vi "Velmex cfg simulation.vi"(8 "error in (no error)":errorcluster {"code" format="%.0x"}, 10 "Channel parsed command info":T1, 11 "input cluster":refnum<class "VelmexStage.lvclass">) -> (0 "error out":errorcluster, 2 "new commands":string, 3 "output cluster":refnum<class "VelmexStage.lvclass">)   [LabVIEW 2013, in "VelmexStage.lvclass"]
uses:
  VelmexStage.lvclass
  channel parsed cmd cluster.ctl
  VelmexStage.lvclass/VelmexStage.ctl
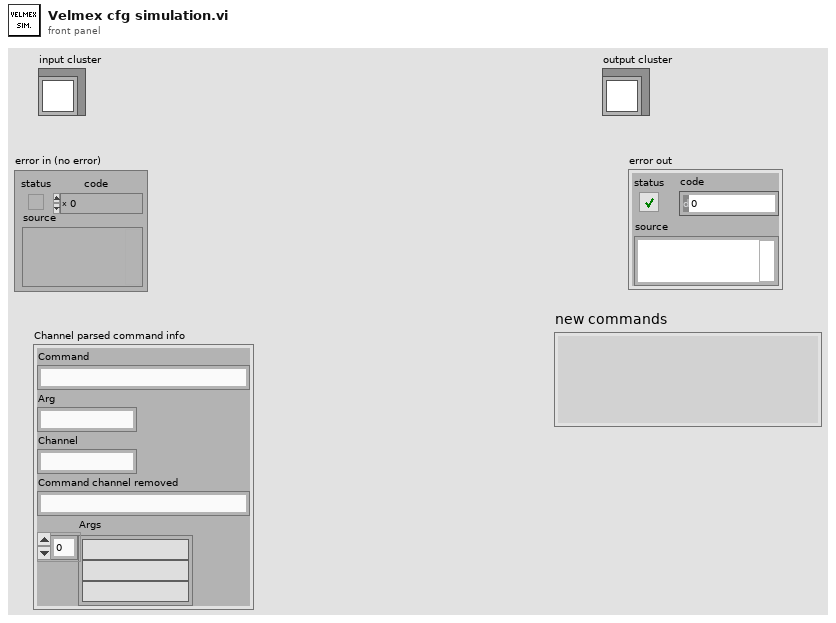
[diagram p1: front panel]
types:
  T1 = typedef "channel parsed cmd cluster.ctl" = cluster{"Command":string, "Arg":string, "Channel":string, "Command channel removed":string, "Args":string[]}
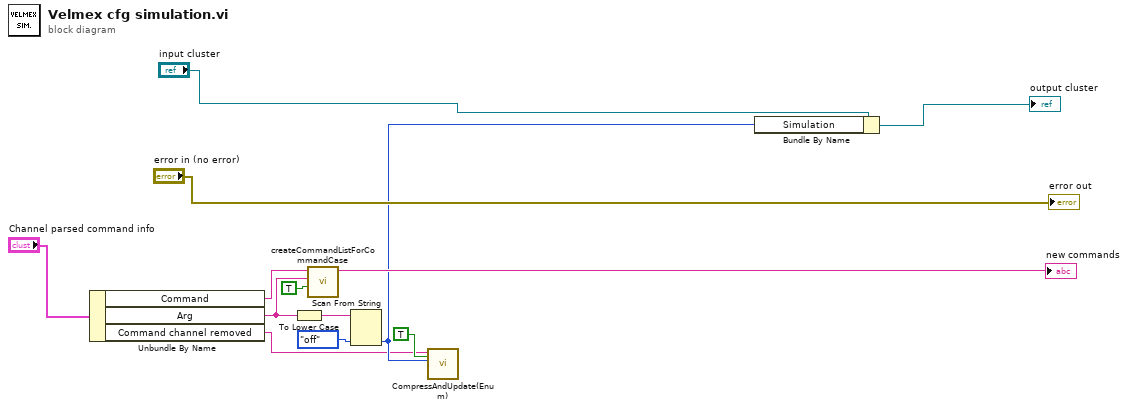
[diagram p0: block diagram]
diagram:
  n1 = Unbundle By Name("Channel parsed command info") -> ("Command"=w2:string, "Arg"=w5:string, "Command channel removed"=w1:string)
  n2 = To Lower Case(string=w5) -> (all lower case string=w7:string)
  n3 = call "createCommandListForCommandCase.vi"("immediate Check (only once)"=TRUE, "setvalue"=w5, "command"=w2) -> ("new commands"=→"new commands":string)  [unwired: 8 in]
  n4 = Scan From String(input string=w7, default 1=enum16{"off", "on"}."off") -> (output 1=w3:enum16{"off", "on"})  [unwired: 3 in, 3 out]
  n5 = call "CompressAndUpdate(Enum).vi"("force CVT update (false)"=TRUE ("force CVT update"), "enum variant"=w3, "command or variable name"=w1) -> ()  [unwired: 8 in, 1 out]
  n6 = Bundle By Name(cluster="input cluster", "Simulation"=w3) -> (→"output cluster":refnum<class "VelmexStage.lvclass">)
  "error out" <- "error in (no error)"
